vi "VG_BT3564.vi"() -> ()   [LabVIEW 2020]
panel:
  out "BT3564":string
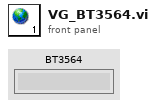
[diagram p1: front panel]
diagram:
